vi "Process-received-message.vi"(7 "Data ref in":T1, 8 "error in (no error)":errorcluster, 10 "Message":refnum<class "Message.lvclass">, 11 "Client in":T2) -> (0 "error out":errorcluster, 3 "Client out":T2, 5 "Data ref out":T1)   [LabVIEW 2013, in "PowderDeposition.lvlib" / "PD-Main.lvclass"]
doc: "This function wraps the message checks, analysis and response action functions.\nThe validity of the message and message origin is checked, after which the appropriate module action is determined and executed.\n\nThe actions should be implemented by the module integrator."
uses:
  Main/PD-Main.lvclass
  Object-reference.ctl
  PD-Client.lvclass
  SA-SLMAPI/Sources/Message.lvclass
  Main/Object-reference.ctl
  SA-SLMAPI/Sources/Message.lvclass/Message.ctl
  Main/PD-Main.lvclass/PD-Main.ctl
  SA-SLMAPI/Sources/Load-settings/Load-settings.lvclass
  Main/PD-actions.ctl
  SA-SLMAPI/Sources/Load-settings/Load-settings.lvclass/Load-settings.ctl
  SA-SLMAPI/Sources/Load-file/Load-file.lvclass
  SA-SLMAPI/Sources/Load-file/Load-file.lvclass/Load-file.ctl
  Main/Enqueue-modes.ctl
  Main/Read Status.vi
  Main/Write Path.vi
  SA-SLMAPI/Sources/Send-status/Send-status.lvclass
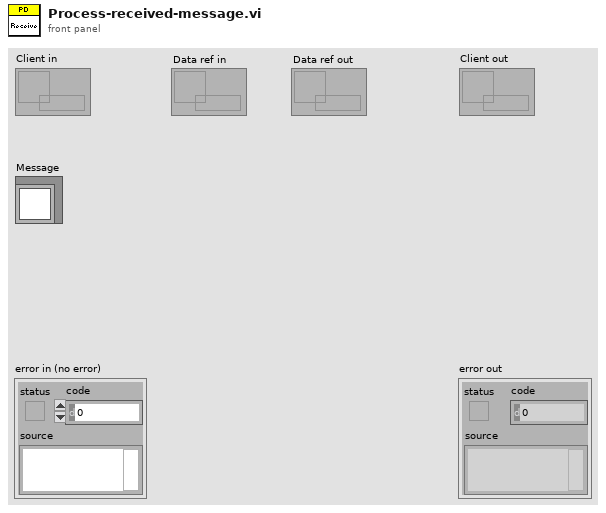
[diagram p1: front panel]
types:
  T1 = typedef "PowderDeposition.lvlib/PD-Main.lvclass/Object-reference.ctl" = refnum<data-value>
  T2 = typedef "PowderDeposition.lvlib/PD-Client.lvclass/Object-reference.ctl" = refnum<data-value>
  T3 = typedef "PowderDeposition.lvlib/PD-Main.lvclass/Enqueue-modes.ctl" = enum16{"Default", "Priority", "Flush"}
  T4 = typedef "PowderDeposition.lvlib/PD-Client.lvclass/Supported-messages.ctl" = enum16{"Heartbeat", "Error", "Client stopped", "Action", "Query status", "Send status", "Get clients"}
  T5 = typedef "PowderDeposition.lvlib/PD-Client.lvclass/Supported-modules.ctl" = enum16{"Server", "All", "SLMControl", "PowderDeposition", "StrategyParser", "CameraVision", "MaterialCharacterization", "StatusMonitor", "SLMSimulation", "LaserCharacterization"}
  T6 = typedef "PowderDeposition.lvlib/PD-Data.lvclass/Statusses.ctl" = enum16{"Idle", "Initialized", "Configured", "Activated", "Started", "Paused", "Stopped", "Reset", "Error", "Exited"}
  T7 = typedef "PowderDeposition.lvlib/PD-Client.lvclass/Supported-actions.ctl" = enum16{"Load settings", "Load file", "Activate", "Start", "Stop", "Reset", "Exit"}
  T8 = typedef "PowderDeposition.lvlib/PD-Main.lvclass/PD-actions.ctl" = enum16{"Idle", "Initialize", "Signal initialized", "Activate all motors", "Deactivate all motors", "Update motor activity", "Update selected motor", "Update motor status", "Update selected sequence", "Load sequences with dialog", "Load sequences from file", "Save sequences", "Add to sequence", "Remove from sequence", "Clear sequences", "Update available actions", "Create action", "Edit action", "Execute action", "Execute sequences", "Execute seq with assert", "Abort", "Exit"}
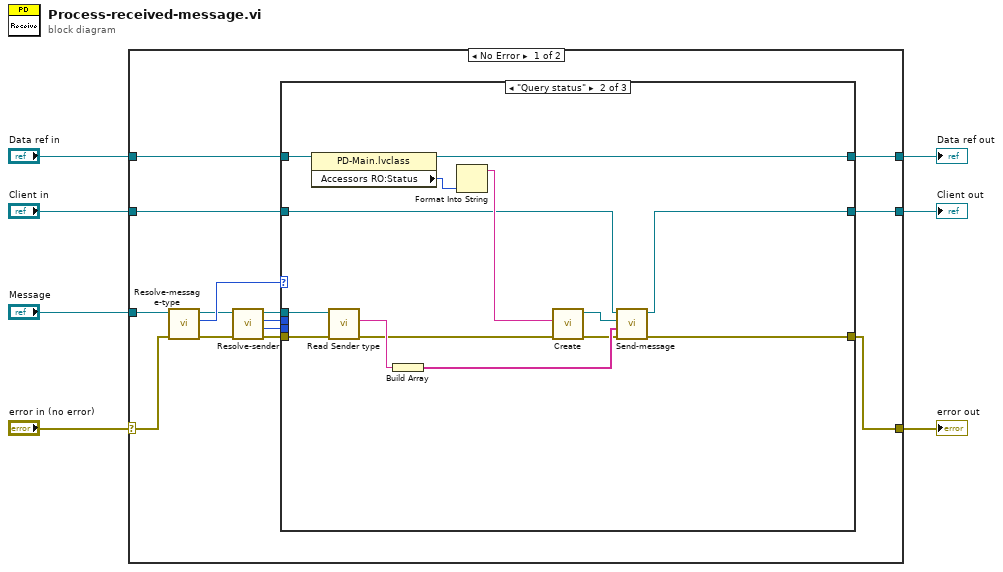
[diagram p0: block diagram]
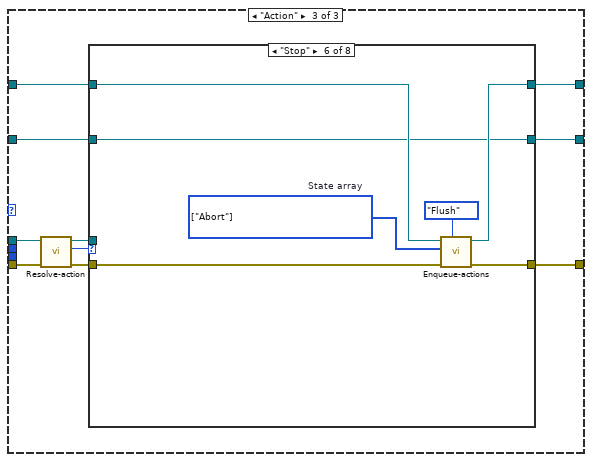
[diagram p3: hidden frame]
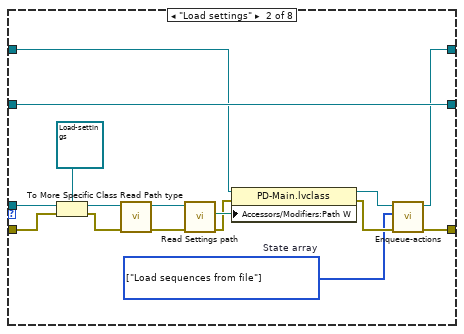
[diagram p5: hidden frame]
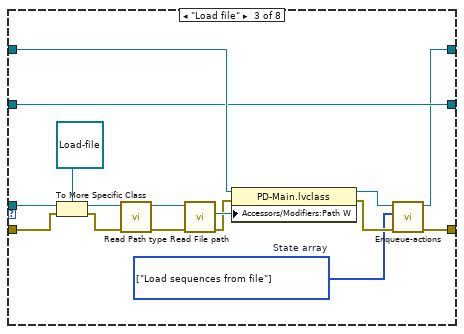
[diagram p6: hidden frame]
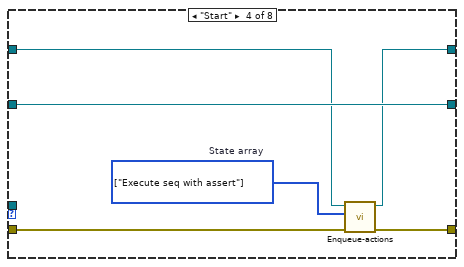
[diagram p7: hidden frame]
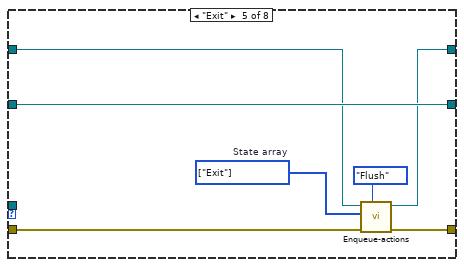
[diagram p8: hidden frame]
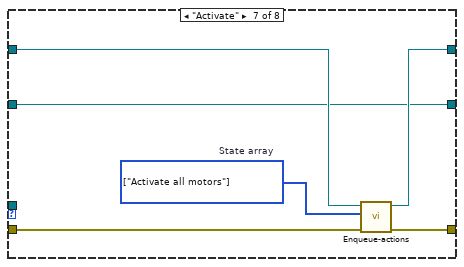
[diagram p9: hidden frame]
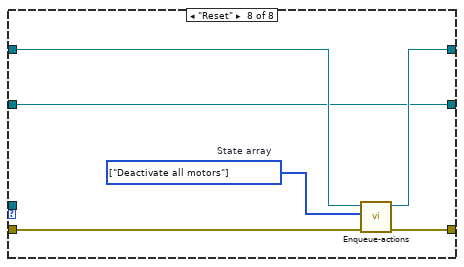
[diagram p10: hidden frame]
diagram:
  n1 = case shown="No Error" "error in (no error)" {
    selector: "error in (no error)" -> [w19 w118]
    tunnel: [w8 w118] -> w6
    tunnel: [w20 w117] -> w4
    tunnel: "Client in" -> [w21 w117]
    tunnel: "Message" -> [w18 _]
    tunnel: "Data ref in" -> [w10 w116]
    tunnel: [w9 w116] -> w1
    frame No Error {
      n2 = call "Resolve-message-type.vi"("error in (no error)"=w19, "Message"=w18) -> ("error out"=w15:errorcluster, "Message type"=w17:T4, "Message dup"=w16:refnum<class "Message.lvclass">)  [unwired: 7 in]
      n3 = call "Resolve-sender.vi"("error in (no error)"=w15, "Message"=w16) -> ("error out"=w12:errorcluster, "Sender ID"=w13:i32, "Sender type"=w14:T5, "Message dup"=w11:refnum<class "Message.lvclass">)  [unwired: 6 in]
      n4 = case shown="\"Query status\"" w17 {
        tunnel: [w23 w25 w39] -> w8
        tunnel: w21 -> [w24 w28 w47]
        tunnel: [w24 w27 w45] -> w20
        tunnel: w14 -> [_ _ _]
        tunnel: w13 -> [_ _ _]
        tunnel: w12 -> [w23 w36 w41]
        tunnel: w11 -> [_ w37 w40]
        tunnel: w10 -> [w22 w38 w48]
        tunnel: [w22 w35 w46] -> w9
        frame Default {
        }
        frame "Query status" {
          n5 = property class="PD-Main.lvclass"(reference=w38) -> (reference out=w35:T1, "Accessors RO:Status"=w34:T6)  [unwired: 1 in, 1 out]
          n6 = call "Read Sender type.vi"("error in (no error)"=w36, "Message in"=w37) -> ("error out"=w30:errorcluster, "Sender type"=w32:string)  [unwired: 7 in, 1 out]
          n7 = Build Array(w32) -> (w31:string[])
          n8 = Format Into String(w34) -> (resulting string=w33:string)  [unwired: 3 in, 1 out]
          n9 = call "Create.vi"("error in (no error)"=w30, "Status"=w33) -> ("error out"=w29:errorcluster, "Send-status out"=w26:refnum<class "Send-status.lvclass">)  [unwired: 8 in]
          n10 = call "Send-message.vi"("error in (no error)"=w29, "Receivers"=w31, "Message"=w26, "Client in"=w28) -> ("error out"=w25:errorcluster, "Client out"=w27:T2)  [unwired: 6 in]
        }
        frame "Action" {
          n11 = call "Resolve-action.vi"("error in (no error)"=w41, "Message"=w40) -> ("error out"=w42:errorcluster, "Action"=w43:T7, "Message dup"=w44:refnum<class "Message.lvclass">)  [unwired: 7 in]
          n12 = case shown="\"Stop\"" w43 {
            tunnel: w48 -> [w51 w54 w70 w86 w91 w100 w107 w113]
            tunnel: w47 -> [w50 w67 w69 w89 w96 w98 w105 w111]
            tunnel: [w51 w53 w68 w87 w92 w99 w106 w112] -> w46
            tunnel: [w50 w67 w69 w89 w96 w98 w105 w111] -> w45
            tunnel: w44 -> [_ w56 w73 _ _ _ _ _]
            tunnel: w42 -> [w49 w55 w72 w85 w90 w97 w104 w110]
            tunnel: [w49 w52 w71 w84 w93 w101 w108 w114] -> w39
            frame Default {
            }
            frame "Load settings" {
              w57 = T8[] [enum."Load sequences from file"] items=["Idle", "Initialize", "Signal initialized", "Activate all motors", "Deactivate all motors", "Update motor activity", "Update selected motor", "Update motor status", "Update selected sequence", "Load sequences with dialog", "Load sequences from file", "Save sequences", "Add to sequence", "Remove from sequence", "Clear sequences", "Update available actions", "Create action", "Edit action", "Execute action", "Execute sequences", "Execute seq with assert", "Abort", "Exit"]  # State array
              n13 = To More Specific Class(target class=refnum<class "Load-settings.lvclass"> refnum ("Messages.lvlib:Load-settings.lvclass"), reference=w56, error in=w55) -> (specific class reference=w65:refnum<class "Load-settings.lvclass">, error out=w64:errorcluster)
              n14 = call "Read Path type.vi"("error in (no error)"=w64, "Load-settings in"=w65) -> ("error out"=w63:errorcluster, "Load-settings out"=w62:refnum<class "Load-settings.lvclass">)  [unwired: 7 in, 1 out]
              n15 = call "Read Settings path.vi"("error in (no error)"=w63, "Load-settings in"=w62) -> ("error out"=w60:errorcluster, "Settings path"=w61:path)  [unwired: 7 in, 1 out]
              n16 = property class="PD-Main.lvclass"(reference=w54, error in=w60, "Accessors/Modifiers:Path W"=w61) -> (reference out=w59:T1, error out=w58:errorcluster)
              n17 = call "Enqueue-actions.vi"("error in (no error)"=w58, "State array"=w57, "State queue in"=w59) -> ("error out"=w52:errorcluster, "State queue out"=w53:T1)  [unwired: 6 in, 1 out]
            }
            frame "Load file" {
              w74 = T8[] [enum."Load sequences from file"] items=["Idle", "Initialize", "Signal initialized", "Activate all motors", "Deactivate all motors", "Update motor activity", "Update selected motor", "Update motor status", "Update selected sequence", "Load sequences with dialog", "Load sequences from file", "Save sequences", "Add to sequence", "Remove from sequence", "Clear sequences", "Update available actions", "Create action", "Edit action", "Execute action", "Execute sequences", "Execute seq with assert", "Abort", "Exit"]  # State array
              n18 = To More Specific Class(target class=refnum<class "Load-file.lvclass"> refnum ("Messages.lvlib:Load-file.lvclass"), reference=w73, error in=w72) -> (specific class reference=w82:refnum<class "Load-file.lvclass">, error out=w81:errorcluster)
              n19 = call "Read Path type.vi"("error in (no error)"=w81, "Load-file in"=w82) -> ("error out"=w80:errorcluster, "Load-file out"=w79:refnum<class "Load-file.lvclass">)  [unwired: 7 in, 1 out]
              n20 = call "Read File path.vi"("error in (no error)"=w80, "Load-file in"=w79) -> ("error out"=w77:errorcluster, "File path"=w78:path)  [unwired: 7 in, 1 out]
              n21 = property class="PD-Main.lvclass"(reference=w70, error in=w77, "Accessors/Modifiers:Path W"=w78) -> (reference out=w76:T1, error out=w75:errorcluster)
              n22 = call "Enqueue-actions.vi"("error in (no error)"=w75, "State array"=w74, "State queue in"=w76) -> ("error out"=w71:errorcluster, "State queue out"=w68:T1)  [unwired: 6 in, 1 out]
            }
            frame "Start" {
              w88 = T8[] [enum."Execute seq with assert"] items=["Idle", "Initialize", "Signal initialized", "Activate all motors", "Deactivate all motors", "Update motor activity", "Update selected motor", "Update motor status", "Update selected sequence", "Load sequences with dialog", "Load sequences from file", "Save sequences", "Add to sequence", "Remove from sequence", "Clear sequences", "Update available actions", "Create action", "Edit action", "Execute action", "Execute sequences", "Execute seq with assert", "Abort", "Exit"]  # State array
              n23 = call "Enqueue-actions.vi"("error in (no error)"=w85, "State array"=w88, "State queue in"=w86) -> ("error out"=w84:errorcluster, "State queue out"=w87:T1)  [unwired: 6 in, 1 out]
            }
            frame "Exit" {
              w95 = T8[] [enum."Exit"] items=["Idle", "Initialize", "Signal initialized", "Activate all motors", "Deactivate all motors", "Update motor activity", "Update selected motor", "Update motor status", "Update selected sequence", "Load sequences with dialog", "Load sequences from file", "Save sequences", "Add to sequence", "Remove from sequence", "Clear sequences", "Update available actions", "Create action", "Edit action", "Execute action", "Execute sequences", "Execute seq with assert", "Abort", "Exit"]  # State array
              n24 = call "Enqueue-actions.vi"("Enqueue mode"=Enqueue-modes."Flush", "error in (no error)"=w90, "State array"=w95, "State queue in"=w91) -> ("error out"=w93:errorcluster, "State queue out"=w92:T1)  [unwired: 5 in, 1 out]
            }
            frame "Stop" {
              w103 = T8[] [enum."Abort"] items=["Idle", "Initialize", "Signal initialized", "Activate all motors", "Deactivate all motors", "Update motor activity", "Update selected motor", "Update motor status", "Update selected sequence", "Load sequences with dialog", "Load sequences from file", "Save sequences", "Add to sequence", "Remove from sequence", "Clear sequences", "Update available actions", "Create action", "Edit action", "Execute action", "Execute sequences", "Execute seq with assert", "Abort", "Exit"]  # State array
              n25 = call "Enqueue-actions.vi"("Enqueue mode"=Enqueue-modes."Flush", "error in (no error)"=w97, "State array"=w103, "State queue in"=w100) -> ("error out"=w101:errorcluster, "State queue out"=w99:T1)  [unwired: 5 in, 1 out]
            }
            frame "Activate" {
              w109 = T8[] [enum."Activate all motors"] items=["Idle", "Initialize", "Signal initialized", "Activate all motors", "Deactivate all motors", "Update motor activity", "Update selected motor", "Update motor status", "Update selected sequence", "Load sequences with dialog", "Load sequences from file", "Save sequences", "Add to sequence", "Remove from sequence", "Clear sequences", "Update available actions", "Create action", "Edit action", "Execute action", "Execute sequences", "Execute seq with assert", "Abort", "Exit"]  # State array
              n26 = call "Enqueue-actions.vi"("error in (no error)"=w104, "State array"=w109, "State queue in"=w107) -> ("error out"=w108:errorcluster, "State queue out"=w106:T1)  [unwired: 6 in, 1 out]
            }
            frame "Reset" {
              w115 = T8[] [enum."Deactivate all motors"] items=["Idle", "Initialize", "Signal initialized", "Activate all motors", "Deactivate all motors", "Update motor activity", "Update selected motor", "Update motor status", "Update selected sequence", "Load sequences with dialog", "Load sequences from file", "Save sequences", "Add to sequence", "Remove from sequence", "Clear sequences", "Update available actions", "Create action", "Edit action", "Execute action", "Execute sequences", "Execute seq with assert", "Abort", "Exit"]  # State array
              n27 = call "Enqueue-actions.vi"("error in (no error)"=w110, "State array"=w115, "State queue in"=w113) -> ("error out"=w114:errorcluster, "State queue out"=w112:T1)  [unwired: 6 in, 1 out]
            }
          }
        }
      }
    }
    frame Error {
    }
  }
  "error out" <- w6
  "Client out" <- w4
  "Data ref out" <- w1
